vi "GyroTracker.vi"(4 "Full Speed Angle Diff":dbl=50.0 min=0.0 max=359.99, 8 "Angle Deadband":dbl=1.0 min=0.0 max=5.0 step=0.001, 9 "Gyro Angle":dbl min=0.0 max=359.0 step=0.25, 10 "Target Speed":dbl min=-1.0 max=1.0 step=0.001, 11 "Target Direction (degrees)":dbl) -> (0 "Right Wheel Speed":dbl, 3 "Left Wheel Speed":dbl)   [LabVIEW 2015]
panel:
  out "Clockwise Offset Speed":dbl
  out "Command Speed":dbl
  out "Angle Error":dbl
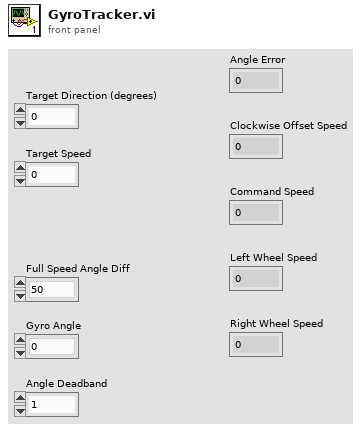
[diagram p1: front panel]
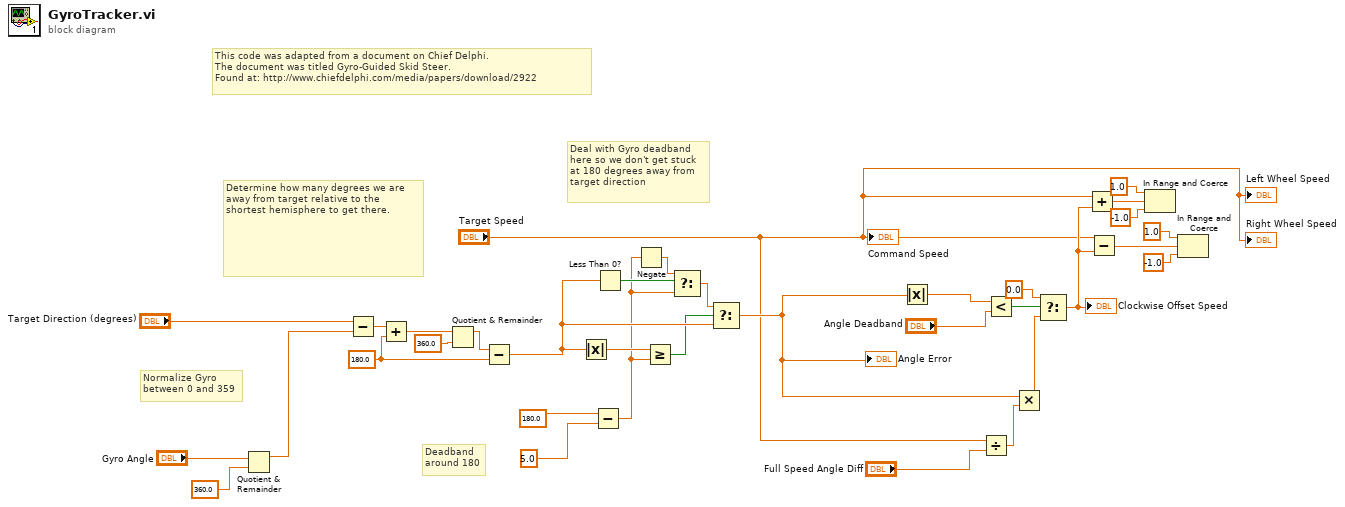
[diagram p0: block diagram]
diagram:
  w29 = 180.0 ("y")
  # "Deadband\naround 180"
  # "Deal with Gyro deadband\nhere so we don't get stuck\nat 180 degrees away from\ntarget direction"
  # "Determine how many degrees we are away from target relative to the shortest hemisphere to get there."
  # "Normalize Gyro\nbetween 0 and 359"
  # "This code was adapted from a document on Chief Delphi.\nThe document was titled Gyro-Guided Skid Steer.\nFound at: http://www.chiefdelphi.com/media/papers/download/2922"
  n1 = Quotient & Remainder(x="Gyro Angle", y=360.0) -> (x-y*floor(x/y)=w15:dbl)  [unwired: 1 out]
  n2 = Subtract(x="Target Direction (degrees)", y=w15) -> (x-y=w33:dbl)
  n3 = Add(x=w33, y=w29) -> (x+y=w32:dbl)
  n4 = Quotient & Remainder(x=w32, y=360.0) -> (x-y*floor(x/y)=w30:dbl)  [unwired: 1 out]
  n5 = Subtract(x=w30, y=w29) -> (x-y=w28:dbl)
  n6 = Absolute Value(x=w28) -> (abs(x)=w13:dbl)
  n7 = Subtract(x=180.0 ("y"), y=5.0) -> (x-y=w7:dbl)
  n8 = Less Than 0?(x=w28) -> (x < 0?=w10:bool)
  n9 = Negate(x=w7) -> (-x=w9:dbl)
  n10 = Greater Or Equal?(x=w13, y=w7) -> (x >= y?=w12:bool)
  n11 = Select(t=w9, s=w10, f=w7) -> (s? t:f=w11:dbl)
  n12 = Select(t=w11, s=w12, f=w28) -> (s? t:f=w5:dbl)
  "Angle Error" <- w5
  n13 = Absolute Value(x=w5) -> (abs(x)=w3:dbl)
  n14 = Divide(x="Target Speed", y="Full Speed Angle Diff") -> (x/y=w6:dbl)
  n15 = Less?(x=w3, y="Angle Deadband") -> (x < y?=w26:bool)
  n16 = Multiply(x=w5, y=w6) -> (x*y=w2:dbl)
  n17 = Select(t=0.0, s=w26, f=w2) -> (s? t:f=w24:dbl)
  "Clockwise Offset Speed" <- w24
  n18 = Add(x="Target Speed", y=w24) -> (x+y=w23:dbl)
  n19 = Subtract(x="Target Speed", y=w24) -> (x-y=w18:dbl)
  n20 = In Range and Coerce(upper limit=1.0, x=w23, lower limit=-1.0) -> ()  [unwired: 2 out]
  n21 = In Range and Coerce(upper limit=1.0, x=w18, lower limit=-1.0) -> ()  [unwired: 2 out]
  "Left Wheel Speed" <- "Target Speed"
  "Right Wheel Speed" <- "Target Speed"
  "Command Speed" <- "Target Speed"
